vi "DebugControl_Provider_OnCommand.vi"(10 "Command ID":string, 11 "objects":T1[](array[typedef])) -> ()   [LabVIEW 2018]
uses:
  <resource>/Framework/Providers/API/ItemRef.ctl
panel:
  out "error out":errorcluster
  in  "error in":errorcluster
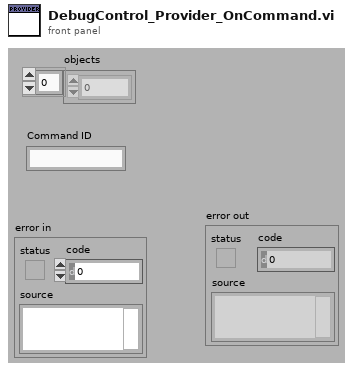
[diagram p1: front panel]
types:
  T1 = typedef "ItemRef.ctl" = u64
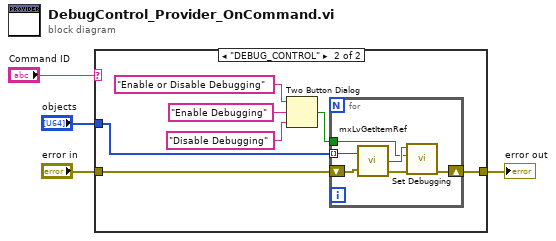
[diagram p0: block diagram]
diagram:
  n1 = case shown="\"DEBUG_CONTROL\"" "Command ID" {
    tunnel: "objects" -> [_ w12]
    tunnel: "error in" -> [w5 w11]
    tunnel: [w5 w10] -> w1
    frame Default {
    }
    frame "DEBUG_CONTROL" {
      n2 = Two Button Dialog(message="Enable or Disable Debugging" ("string"), 1:"Disable Debugging" ("F button name (\"Cancel\")"), 2:"Enable Debugging" ("T button name (\"OK\")")) -> (T button?=w7:bool)
      n3 = for {
        tunnel: w12 -> [w18] mode=indexing
        shift-right: [w14] -> w10
        shift-left: w11 -> [w17]
        tunnel: w7 -> [w13]
        n4 = call <resource>:"mxLvGetItemRef.vi"("Item"=w18, "error in"=w17) -> ("Item Refnum"=w16:refnum<vi>, "error out"=w15:errorcluster)  [unwired: 1 out]
        n5 = call "Set Debugging.vi"("error in (no error)"=w15, "Debugging Control"=w13, "ProjectItem in"=w16) -> ("error out"=w14:errorcluster)  [unwired: 8 in]
      }
    }
  }
  "error out" <- w1
